vi "lvpeak_start_acquisition.vi"(8 "error in (no error)":errorcluster, 11 "camera_id":u64) -> (0 "error out":errorcluster, 3 "camera_id out":u64)   [LabVIEW 2024, in "Vision.lvlib"]
uses:
  Vision.lvlib
  bin/LVPeak.dll
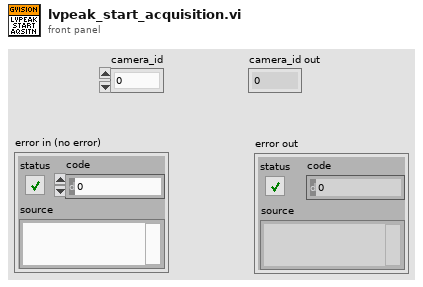
[diagram p1: front panel]
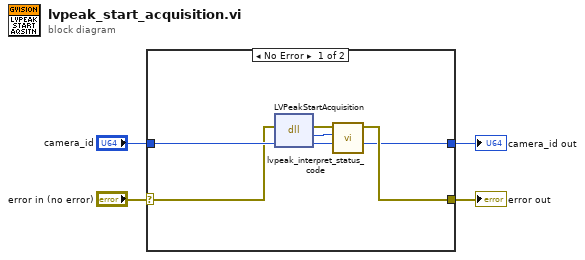
[diagram p0: block diagram]
diagram:
  n1 = case shown="No Error" "error in (no error)" {
    selector: "error in (no error)" -> [w7 w11]
    tunnel: [w6 w11] -> w3
    tunnel: [w5 _] -> w2
    tunnel: "camera_id" -> [w8 _]
    frame No Error {
      n2 = dll-call lib="C:/Users/cfang/Desktop/nebraska-silicon-lab/pixel-gantry-control/Gantry/Shared Components/bin/LVPeak.dll" fn="LVPeakStartAcquisition"(error in=w7, "camera_id"=w8) -> (error out=w10:errorcluster, "return type"=w9:i32, "camera_id"=w5:u64)  [unwired: 2 in, 1 out]
      n3 = call "lvpeak_interpret_status_code.vi"("status_code"=w9, "error in (no error)"=w10) -> ("error out"=w6:errorcluster)  [unwired: 9 in]
    }
    frame Error {
    }
  }
  "error out" <- w3
  "camera_id out" <- w2
